vi "Timer_Start.vi"(11 "in Timer":T1 {"Accumulated TIme" format="%13.5p"; "StartTime" format="%13.5p"}) -> (3 "out Timer":T1 {"Accumulated TIme" format="%13.5p"; "StartTime" format="%13.5p"})   [LabVIEW 2019, in "Trajectory_Library.lvlib"]
doc: "Start the timer running. Just set the running flag to true indicating that all time requests should be relative to the system clock.\n\nInputs:\n - Timer -- The Timer data cluster\n\nOutputs:\n - Timer -- The modified Timer data cluster"
uses:
  Trajectory_Library.lvlib
  TIMER.ctl
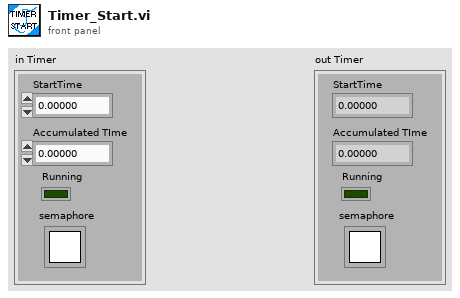
[diagram p1: front panel]
types:
  T1 = typedef "Trajectory_Library.lvlib/TIMER.ctl" = cluster{"StartTime":dbl, "Accumulated TIme":dbl, "Running":bool, "semaphore":T2}
  T2 = typedef "Semaphore RefNum" = refnum<k1>
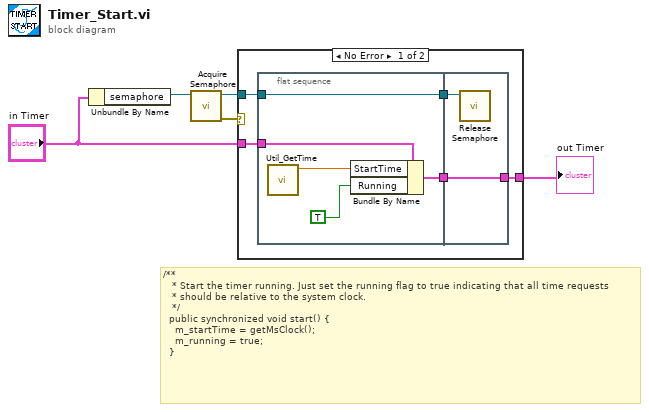
[diagram p0: block diagram]
diagram:
  # "/**\n   * Start the timer running. Just set the running flag to true indicating that all time requests\n   * should be relative to the system clock.\n   */\n  public synchronized void start() {\n    m_startTime = getMsClock();\n    m_running = true;\n  }"
  n1 = Unbundle By Name("in Timer") -> ("semaphore"=w4:T2)
  n2 = call <vilib>:"Acquire Semaphore.vi"("semaphore"=w4) -> ("error out"=w2:errorcluster, "semaphore out"=w1:T2)  [unwired: 4 in, 1 out]
  n3 = case shown="No Error" w2 {
    tunnel: "in Timer" -> [w10 w18]
    tunnel: [w9 w18] -> w5
    tunnel: w1 -> [w6 _]
    frame No Error {
      n4 = flat-sequence {
        tunnel: w10 -> [w15]
        tunnel: [w14] -> w8
        tunnel: [w11] -> w7
        tunnel: w6 -> [w11]
        tunnel: [w17] -> w9
        tunnel: w8 -> [w17]
        tunnel: w7 -> [w16]
        frame #0 {
          n5 = call "Util_GetTime.vi"() -> ("FPGA_Time_Seconds"=w12:dbl)  [unwired: 10 in, 1 out]
          n6 = Bundle By Name(cluster=w15, "StartTime"=w12, "Running"=TRUE) -> (w14:T1)
        }
        frame #1 {
          n7 = call <vilib>:"Release Semaphore.vi"("semaphore"=w16) -> ()  [unwired: 5 in, 2 out]
        }
      }
    }
    frame Error {
    }
  }
  "out Timer" <- w5
